vi "Placos.vi"(2 "Safety Buttons back 2":bool, 3 "Safety Buttons back":bool, 4 "Safety X":bool) -> ()   [LabVIEW 2017]
uses:
  <vilib>/Rock Robotics/WPI/Solenoid/WPI_SolenoidValue.ctl
  Robot Global Data.vi
  <vilib>/Rock Robotics/WPI/Solenoid/WPI_SolenoidSetEnum.vi
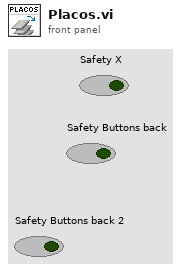
[diagram p1: front panel]
types:
  T1 = typedef "WPI_SolenoidValue.ctl" = enum16{"Off", "On", "Forward", "Reverse"}
  T2 = typedef "WPI_SolenoidDevRef.ctl" = cluster{"DevStatus":errorcluster, "Pneumatics Control Module":u8, "Forward Solenoid Channel":T3, "Reverse Solenoid Channel":T3}
  T3 = typedef "WPI_SolenoidChannel.ctl" = enum8{"Solenoid 0", "Solenoid 1", "Solenoid 2", "Solenoid 3", "Solenoid 4", "Solenoid 5", "Solenoid 6", "Solenoid 7", "Invalid"}
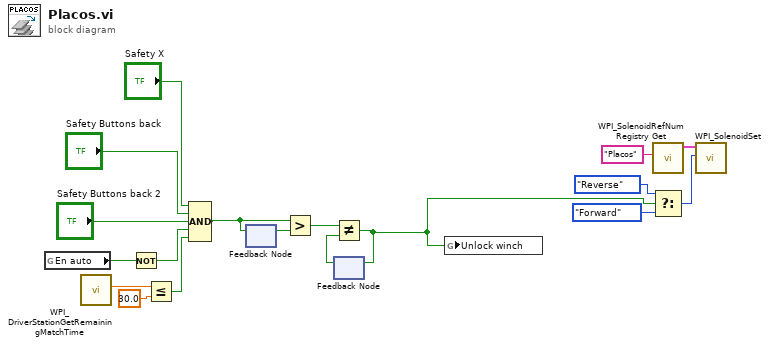
[diagram p0: block diagram]
diagram:
  n1 = global read "Robot Global Data.vi" "En auto"() -> (w18:bool)
  n2 = call <vilib>:"WPI_DriverStationGetRemainingMatchTime.vi"() -> ("Match Time(s)"=w16:sgl)  [unwired: 10 in, 1 out]
  n3 = Not(x=w18) -> (.not. x?=w17:bool)
  n4 = Less Or Equal?(x=w16, y=sgl 30.0) -> (x <= y?=w14:bool)
  n5 = Compound Arithmetic op=AND("Safety X", "Safety Buttons back", "Safety Buttons back 2", w17, w14) -> (w2:bool)
  n6 = feedback #1() -> (w5:bool)  [unwired: 1 in]
  n7 = feedback-in #1(w2) -> ()
  n8 = Greater?(x=w2, y=w5) -> (0:w4:bool)
  n9 = feedback #2() -> (w3:bool)  [unwired: 1 in]
  n10 = Not Equal?(x=w4, y=w3) -> (x != y?=w1:bool)
  n11 = feedback-in #2(w1) -> ()
  n12 = global write "Robot Global Data.vi" "Unlock winch"(w1) -> ()
  n13 = call <vilib>:"WPI_SolenoidRefNum Registry Get.vi"("refnum name"="Placos") -> ("SolenoidDevRef"=w10:T2)  [unwired: 9 in, 1 out]
  n14 = Select(t=WPI_SolenoidValue."Reverse" ("Value"), s=w1, f=WPI_SolenoidValue."Forward" ("Value")) -> (s? t:f=w7:T1)
  n15 = call-poly <vilib>:"WPI_SolenoidSet.vi"("Value"=w7, "SolenoidDevRef"=w10) -> ()  [unwired: 8 in, 2 out]
